vi "archivo labview bueno 2.vi"() -> ()   [LabVIEW 2019]
uses:
  <vilib>/ptbypt/NI_PtbyPt.lvlib
  <vilib>/Utility/file.llb/Write Delimited Spreadsheet (DBL).vi
panel:
  in  "stop 2":bool
  out "x*y":dbl
  out "output variable":dbl
  in  "file path (dialog if empty)":path
  out "Waveform Chart":dbl(graph)
  in  "frequency":dbl=1.0 format="%0.2f"
  in  "stop":bool
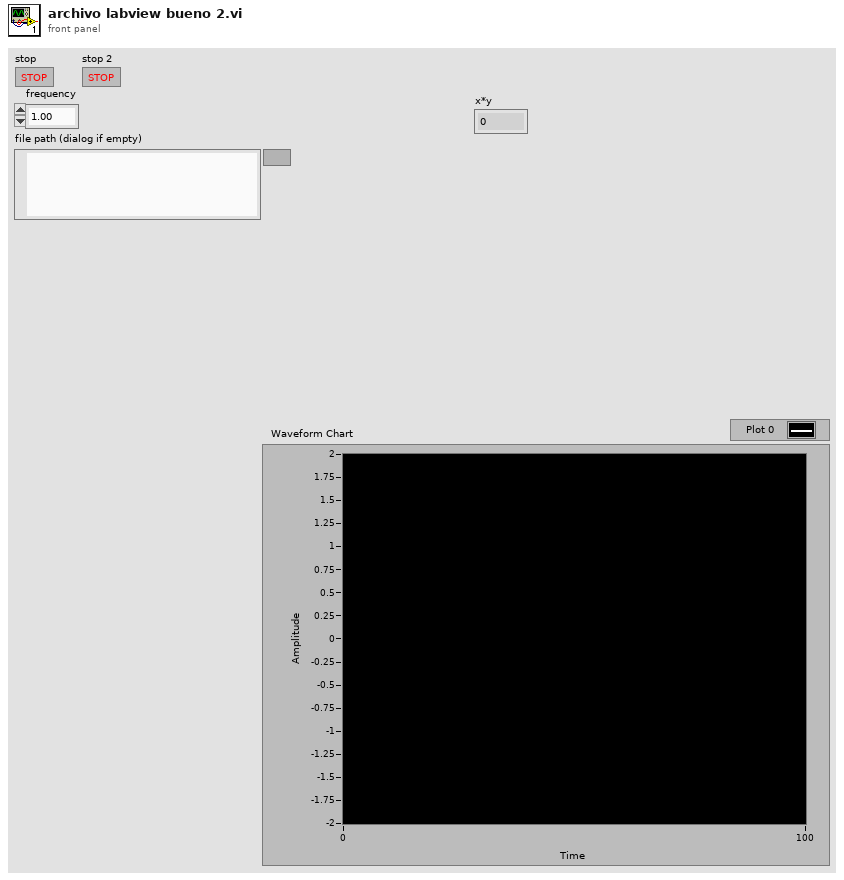
[diagram p1: front panel]
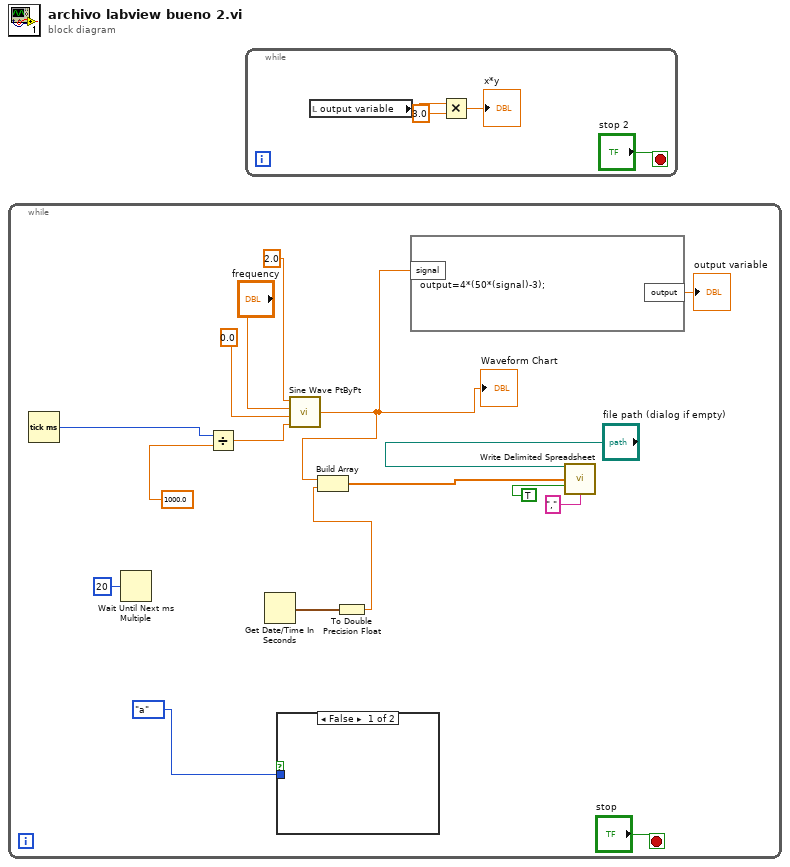
[diagram p0: block diagram]
diagram:
  n1 = while {
    stop <- "stop" stop-if-true
    n2 = Tick Count (ms)() -> (millisecond timer value=w12:u32)
    n3 = Wait Until Next ms Multiple(millisecond multiple=u32 20) -> ()  [unwired: 1 out]
    n4 = Divide(x=w12, y=1000.0) -> (x/y=w11:dbl)
    n5 = Get Date/Time In Seconds() -> (seconds since 1Jan1904=w6:timestamp)
    n6 = case shown="False" {
      selector: _ -> [_ _]
      tunnel: enum16{"", "a", "b", "c"}."a" -> [_ _]
      frame False {
      }
      frame True {
      }
    }
    n7 = call <vilib>:"Sine Wave PtByPt.vi"("time"=w11, "phase"=0.0, "frequency"="frequency", "amplitude"=2.0) -> ("sine wave"=w3:dbl)
    "Waveform Chart" <- w3
    n8 = To Double Precision Float(number=w6) -> (double precision float=w4:dbl)
    n9 = Build Array(w3, w4) -> (w8:dbl[])
    n10 = formula code="output=4*(50*(signal)-3);"("signal"=w3) -> ("output"=→"output variable":dbl)
    n11 = call-poly <vilib>:"Write Delimited Spreadsheet.vi"("file path (dialog if empty)"="file path (dialog if empty)", "1D data"=w8, "append to file? (new file:F)"=TRUE, "delimiter (\\t)"="," ("delimiter (\\t)")) -> ()  [unwired: 10 in, 2 out]
  }
  n12 = while {
    stop <- "stop 2" stop-if-true
    n13 = local read "output variable"() -> (w21:dbl)
    n14 = Multiply(x=w21, y=3.0) -> (x*y=→"x*y":dbl)
  }
